vi "Thorlabs-Update pDataBuffer.vi"(11 "LSM Settings":T1={"Channel Selection"=enum."A", "Pixel Count"={"Pixels in X"=512, "Pixels in Y"=512}, "Field Size"=90.0, "Frames"=2, "Averaging"=FALSE, "Alignment"=0.0, "Scan Mode"=TRUE, "Gain"={"Gain A"=1, "Gain B"=1}, "Enable PMTs"={"A"=TRUE, "B"=TRUE}, "Voltage Range"={"Range A"=10, "Range B"=10}, "Multi Frame Count"=0.0, "Trigger Mode"=2.0, "Real Time Averaging"=TRUE, "Field Size in um"=0.0, "MicronsPerPx"=0.0} {"Field Size" min=5.0 max=255.0 step=1.0 scale=5.0..255.0; "Field Size in um" min=1.0 max=300.0 step=0.1; "MicronsPerPx" min=0.01 step=0.01 format="%.2f"; "Gain"."Gain B" min=1 max=100 step=1; "Gain"."Gain A" min=1 max=100 step=1; "Voltage Range"."Range B" items=["100mV"=5, "200mV"=6, "400mV"=7, "1V"=10, "2V"=11, "4V"=12]; "Voltage Range"."Range A" items=["100mV"=5, "200mV"=6, "400mV"=7, "1V"=10, "2V"=11, "4V"=12]; "Pixel Count"."Pixels in Y" items=["32"=32, "64"=64, "128"=128, "256"=256, "512"=512, "1024"=1024, "2048"=2048]; "Pixel Count"."Pixels in X" items=["32"=32, "64"=64, "128"=128, "256"=256, "512"=512, "1024"=1024, "2048"=2048]}) -> (0 "New pDataBuffer":u16[](array[numeric]), 3 "LSM Settings out":T1={"Channel Selection"=enum."A", "Pixel Count"={"Pixels in X"=512, "Pixels in Y"=512}, "Field Size"=90.0, "Frames"=2, "Averaging"=FALSE, "Alignment"=0.0, "Scan Mode"=TRUE, "Gain"={"Gain A"=1, "Gain B"=1}, "Enable PMTs"={"A"=TRUE, "B"=TRUE}, "Voltage Range"={"Range A"=10, "Range B"=10}, "Multi Frame Count"=0.0, "Trigger Mode"=2.0, "Real Time Averaging"=TRUE, "Field Size in um"=0.0, "MicronsPerPx"=0.0} {"Field Size" min=5.0 max=255.0 step=1.0 scale=5.0..255.0; "Field Size in um" min=1.0 max=300.0 step=0.1; "MicronsPerPx" min=0.01 step=0.01 format="%.2f"; "Gain"."Gain B" min=1 max=100 step=1; "Gain"."Gain A" min=1 max=100 step=1; "Voltage Range"."Range B" items=["100mV"=5, "200mV"=6, "400mV"=7, "1V"=10, "2V"=11, "4V"=12]; "Voltage Range"."Range A" items=["100mV"=5, "200mV"=6, "400mV"=7, "1V"=10, "2V"=11, "4V"=12]; "Pixel Count"."Pixels in Y" items=["32"=32, "64"=64, "128"=128, "256"=256, "512"=512, "1024"=1024, "2048"=2048]; "Pixel Count"."Pixels in X" items=["32"=32, "64"=64, "128"=128, "256"=256, "512"=512, "1024"=1024, "2048"=2048]})   [LabVIEW 2020]
uses:
  _Controls/Confocal Controls.ctl
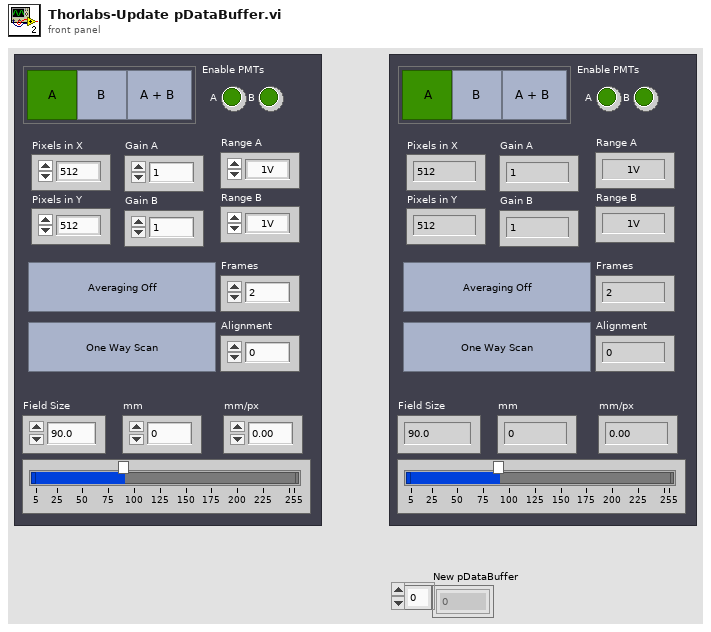
[diagram p1: front panel]
types:
  T1 = typedef "Confocal Controls.ctl" = cluster{"Channel Selection":enum32{"A", "B", "AB"}, "Pixel Count":cluster{"Pixels in X":u32, "Pixels in Y":u32}, "Field Size":dbl, "Frames":u8, "Averaging":bool, "Alignment":dbl, "Scan Mode":bool, "Gain":cluster{"Gain A":u8, "Gain B":u8}, "Enable PMTs":cluster{"A":bool, "B":bool}, "Voltage Range":cluster{"Range A":u16, "Range B":u16}, "Multi Frame Count":dbl, "Trigger Mode":dbl, "Real Time Averaging":bool, "Field Size in um":dbl, "MicronsPerPx":dbl}
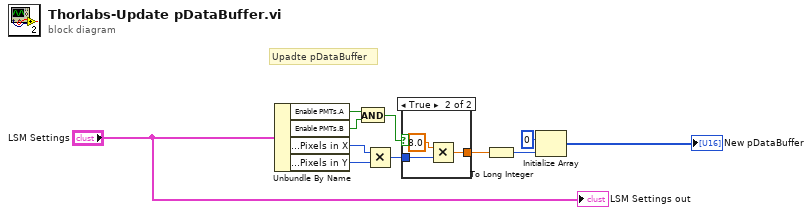
[diagram p0: block diagram]
diagram:
  # "Upadte pDataBuffer"
  n1 = Unbundle By Name("LSM Settings") -> ("Enable PMTs.A"=w10:bool, "Enable PMTs.B"=w9:bool, "Pixel Count.Pixels in X"=w8:u32, "Pixel Count.Pixels in Y"=w7:u32)
  n2 = And(x=w10, y=w9) -> (x .and. y?=w3:bool)
  n3 = Multiply(x=w8, y=w7) -> (x*y=w6:u32)
  n4 = case shown="True" w3 {
    tunnel: w6 -> [w12 w15]
    tunnel: [w12 w13] -> w4
    frame False {
    }
    frame True {
      n5 = Multiply(x=8.0, y=w15) -> (x*y=w13:dbl)
    }
  }
  n6 = To Long Integer(number=w4) -> (32bit integer=w11:i32)
  n7 = Initialize Array(u16 0, w11) -> (→"New pDataBuffer":u16[])
  "LSM Settings out" <- "LSM Settings"
